vi "Video livestream (TCP SERVER).vi"(1 "TCP/IP port":u16=80, 2 "VideoMode":u32, 3 "Interface name":T1="Travcam") -> (0 "Error Out":errorcluster)   [LabVIEW 2015]
doc: "This VI must be loaded when the camera server starts, and also in the list of exported VIs. This VI is not to run directly."
uses:
  <vilib>/userdefined/High Color/IMAQdx.ctl
  <vilib>/vision/driver/IMAQdx.llb/IMAQdx Camera Control Mode.ctl
  <vilib>/vision/driver/NI_Vision_Acquisition_Software.lvlib
  <resource>/objmgr/imaqdx.rc
panel:
  in  "Stop":bool
  out "Video":T2(plugin-control)
  # "PN 25/08/2015"
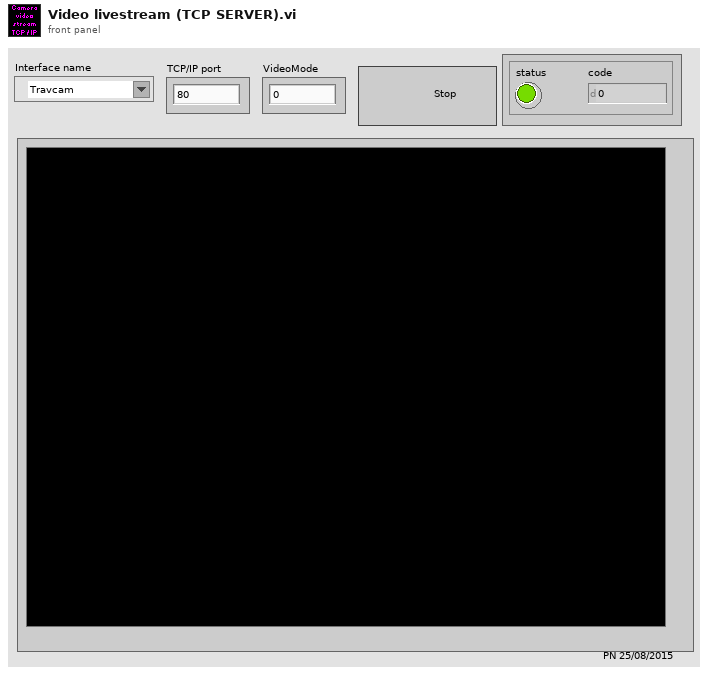
[diagram p1: front panel]
types:
  T1 = typedef "IMAQdx.ctl" = refnum<k21>
  T2 = typedef "IMAQ Image.ctl" = refnum<image>
  T3 = typedef "NI_Vision_Acquisition_Software.lvlib/IMAQdx Camera Control Mode.ctl" = enum32{"Controller", "Listener"}
  T4 = typedef "Image Type" = u32
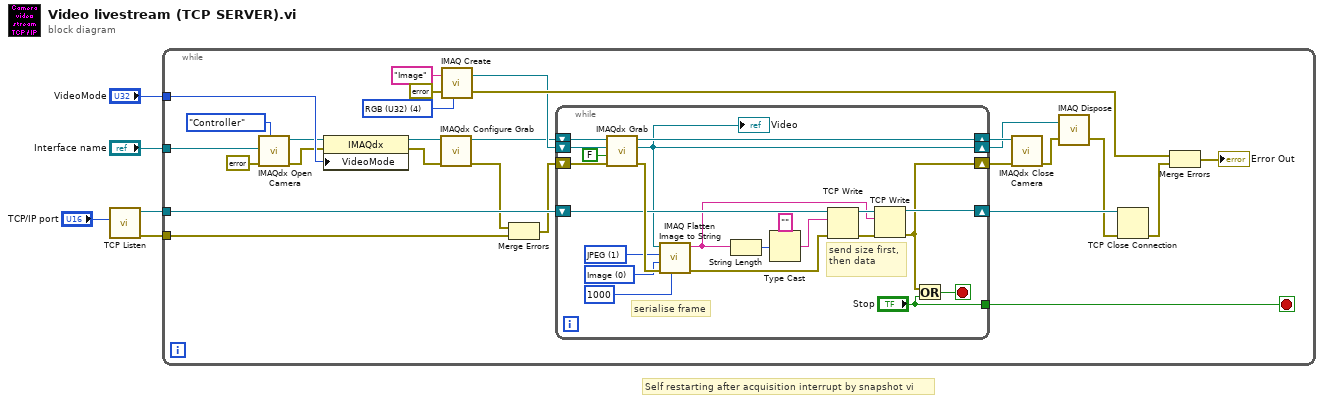
[diagram p0: block diagram]
diagram:
  # "Self restarting after acquisition interrupt by snapshot vi"
  n1 = call <vilib>:"TCP Listen.vi"("port"="TCP/IP port") -> ("error out"=w2:errorcluster, "connection ID"=w3:refnum<k5>)  [unwired: 6 in, 3 out]
  n2 = while {
    tunnel: "VideoMode" -> [w22]
    tunnel: "Interface name" -> [w17]
    tunnel: w2 -> [w11]
    tunnel: w3 -> [w12]
    stop <- w15 stop-if-true
    w30 = T4 4 items=["Grayscale (U8)", "Grayscale (I16)", "Grayscale (SGL)", "Complex (CSG)", "RGB (U32)", "HSL (U32)", "RGB (U64)", "Grayscale (U16)"] ("Image Type")
    n3 = call <vilib>:"IMAQdx Open Camera.vi"("Camera Control Mode"=IMAQdx_Camera_Control_Mode."Controller", "error in"=errorcluster {"status"=FALSE, "code"=0, "source"=""}, "Session In"=w17) -> ("error out"=w19:errorcluster, "Session Out"=w16:T1)  [unwired: 7 in]
    n4 = property class="IMAQdx"(reference=w16, error in=w19, "VideoMode"=w22) -> (reference out=w20:T1, error out=w18:errorcluster)
    n5 = call <vilib>:"IMAQdx Configure Grab.vi"("error in"=w18, "Session In"=w20) -> ("error out"=w10:errorcluster, "Session Out"=w21:T1)  [unwired: 8 in]
    n6 = call "IMAQ Create"("Image Name"="Image", "Image Type"=w30, "error in (no error)"=errorcluster {"status"=FALSE, "code"=0, "source"=""} ("error in")) -> ("New Image"=w28:T2, "error out"=w29:errorcluster)  [unwired: 2 in]
    n7 = Merge Errors(w10, w11) -> (w9:errorcluster)
    n8 = while {
      shift-right: [w52] -> w27
      shift-left: w21 -> [w54]
      shift-right: [w33] -> w24
      shift-left: w28 -> [w53]
      shift-right: [w35] -> w26
      shift-left: w9 -> [w51]
      tunnel: ["Stop"] -> w15
      shift-right: [w36] -> w8
      shift-left: w12 -> [w41]
      stop <- w49 stop-if-true
      w44 = 1 items=["None", "JPEG", "PACKED BINARY"] ("Compression (None)")
      w45 = 0 items=["Image", "Image and Vision Info", "Reference to Image"] ("Type of Flatten (Image and Vision Info)")
      # "serialise frame"
      # "send size first, then data"
      n9 = call <vilib>:"IMAQdx Grab.vi"("error in"=w51, "Wait for Next Buffer? (Yes)"=FALSE, "Image In"=w53, "Session In"=w54) -> ("error out"=w46:errorcluster, "Image Out"=w33:T2, "Session Out"=w52:T1)  [unwired: 4 in, 1 out]
      "Video" <- w33
      n10 = call "IMAQ Flatten Image to String"("Quality (750)"=1000, "error in (no error)"=w46, "Type of Flatten (Image and Vision Info)"=w45, "Compression (None)"=w44, "Image"=w33) -> ("error out"=w39:errorcluster, "Data String"=w34:string)  [unwired: 5 in]
      n11 = String Length(string=w34) -> (length=w43:i32)
      n12 = Type Cast(type="", x=w43) -> (*(type *) &x=w40:string)
      n13 = TCP Write(connection ID=w41, data in=w40, error in (no error)=w39) -> (connection ID out=w37:refnum<k5>, error out=w38:errorcluster)  [unwired: 1 in, 1 out]
      n14 = TCP Write(connection ID=w37, data in=w34, error in (no error)=w38) -> (connection ID out=w36:refnum<k5>, error out=w35:errorcluster)  [unwired: 1 in, 1 out]
      n15 = Or(x=w35, y="Stop") -> (x .or. y?=w49:bool)
    }
    n16 = call <vilib>:"IMAQdx Close Camera.vi"("error in"=w26, "Session In"=w27) -> ("error out"=w23:errorcluster)  [unwired: 9 in]
    n17 = call "IMAQ Dispose"("Image"=w24, "error in (no error)"=w23) -> ("error out"=w7:errorcluster)  [unwired: 4 in]
    n18 = TCP Close Connection(connection ID=w8, error in (no error)=w7) -> (error out=w6:errorcluster)  [unwired: 1 in, 1 out]
    n19 = Merge Errors(w29, w6) -> (→"Error Out":errorcluster)
  }
